vi "editConfiguration.vi"(8 "error in (no error)":errorcluster, 11 "ConfigurationThisComponent in":refnum<class "ConfigurationThisComponent.lvclass">) -> (0 "error out":errorcluster, 3 "ConfigurationThisComponent out":refnum<class "ConfigurationThisComponent.lvclass">)   [LabVIEW 2013, in "ConfigurationThisComponent.lvclass"]
uses:
  ConfigurationThisComponent.lvclass
  ConfigurationThisComponent.lvclass/ConfigurationThisComponent.ctl
  <userlib>/Common/ConfigurationEditor/ConfigurationEditor.lvclass
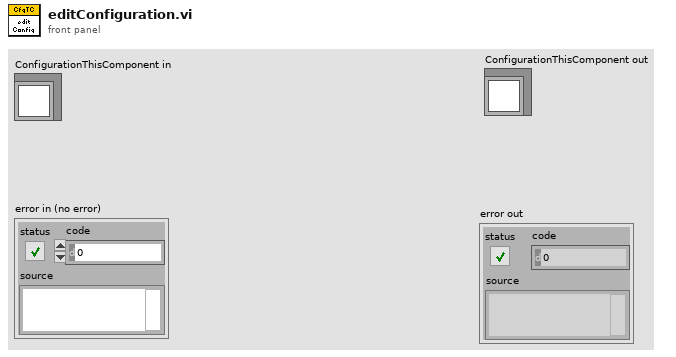
[diagram p1: front panel]
types:
  T1 = enum32{"Bad", "Idle", "Run top level", "Running"}
  T2 = enum32{"Invalid", "Standard", "Closed", "Hidden", "Minimized", "Maximized"}
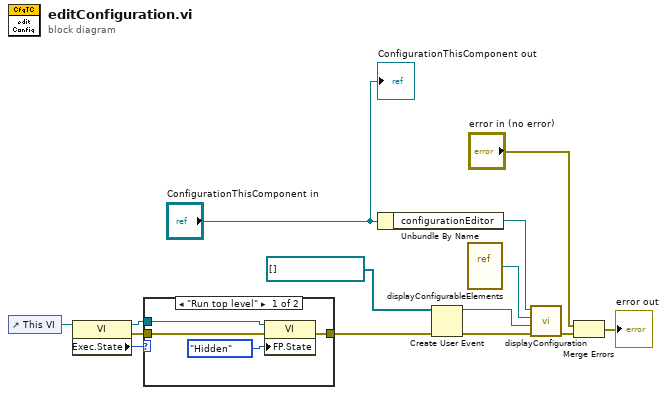
[diagram p0: block diagram]
diagram:
  n1 = control-ref of="This VI"() -> (w10:refnum<vi>)
  n2 = property class="VI"(reference=w10) -> (reference out=w8:refnum<vi>, error out=w6:errorcluster, "Exec.State"=w9:T1)  [unwired: 1 in]
  n3 = case shown="\"Run top level\"" w9 {
    tunnel: w8 -> [w17 _]
    tunnel: [w16 w19] -> w7
    tunnel: w6 -> [w15 w19]
    frame "Run top level" {
      n4 = property class="VI"(reference=w17, error in=w15, "FP.State"=T2."Hidden" ("Front Panel Window:State")) -> (error out=w16:errorcluster)  [unwired: 1 out]
    }
    frame "Running", Default {
    }
  }
  n5 = Unbundle By Name("ConfigurationThisComponent in") -> ("configurationEditor"=w2:refnum<class "ConfigurationEditor.lvclass">)
  n6 = Create User Event(user event datatype=refnum<vi>[] [] ("cfgCtrlRefs"), error in=w7) -> (user event=w12:refnum<user-event>, error out=w11:errorcluster)
  n7 = vi-ref "displayConfigurableElements.vi"() -> (w14:refnum<vi>)
  n8 = call <userlib>:"displayConfiguration.vi"("error in (no error)"=w11, "ctrlRefArrayUsrEvnt"=w12, "configurableElementsVI"=w14, "ConfigurationEditor in"=w2) -> ("error out"=w4:errorcluster)  [unwired: 5 in, 2 out]
  n9 = Merge Errors("error in (no error)", w4) -> (→"error out":errorcluster)
  "ConfigurationThisComponent out" <- "ConfigurationThisComponent in"
